vi "AI_ReadData.vi"(3 "error IO":errorcluster, 4 "count":i32, 6 "Task ID":u32) -> (0 "error out":errorcluster, 1 "data":dbl[](array[numeric]), 2 "Task ID":u32)   [LabVIEW 2015]
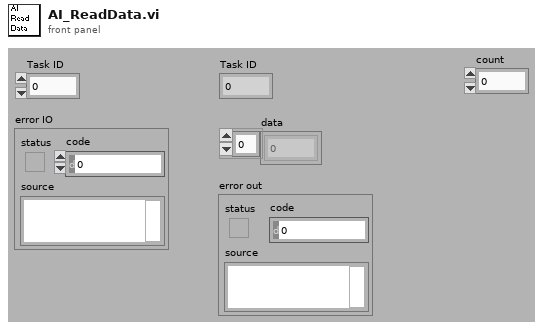
[diagram p1: front panel]
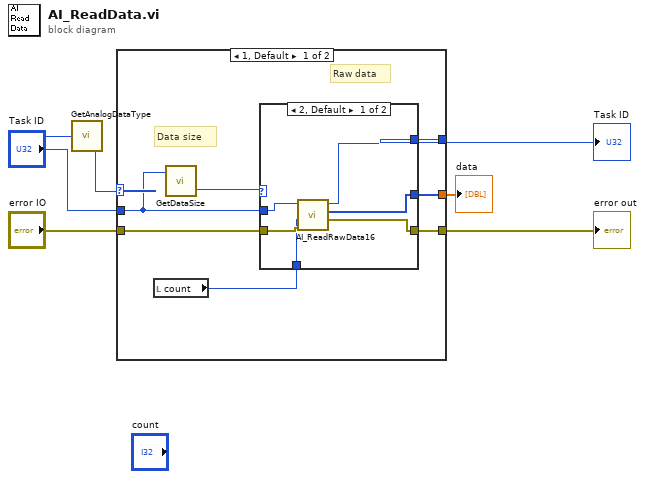
[diagram p0: block diagram]
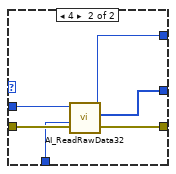
[diagram p2: hidden frame]
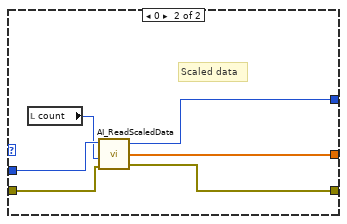
[diagram p3: hidden frame]
diagram:
  n1 = call "GetAnalogDataType.vi"("Task ID"="Task ID") -> ("return type"=w1:i32)
  n2 = case shown="1, Default" w1 {
    tunnel: "Task ID" -> [w8 w31]
    tunnel: "error IO" -> [w13 w30]
    tunnel: [w11 w29] -> w4
    tunnel: [w10 w27] -> w6
    tunnel: [w12 w28] -> w5
    frame 1, Default {
      # "Raw data"
      # "Data size"
      n3 = local read "count"() -> (w9:i32)
      n4 = call "GetDataSize.vi"("Task ID"=w8) -> ("return type"=w7:i32)  [unwired: 2 out]
      n5 = case shown="2, Default" w7 {
        tunnel: w13 -> [w18 w25]
        tunnel: [w17 w24] -> w12
        tunnel: [w16 w23] -> w11
        tunnel: w8 -> [w19 w22]
        tunnel: [w15 w21] -> w10
        tunnel: w9 -> [w14 w20]
        frame 2, Default {
          n6 = call "AI_ReadRawData16.vi"("Task ID"=w19, "count"=w14, "error in (no error)"=w18) -> ("Task ID"=w17:u32, "data"=w15:u16[], "error out"=w16:errorcluster)  [unwired: 1 in, 4 out]
        }
        frame 4 {
          n7 = call "AI_ReadRawData32.vi"("Task ID"=w22, "count"=w20, "error in (no error)"=w25) -> ("Task ID"=w24:u32, "data"=w21:u32[], "error out"=w23:errorcluster)  [unwired: 1 in, 4 out]
        }
      }
    }
    frame 0 {
      # "Scaled data"
      n8 = local read "count"() -> (w26:i32)
      n9 = call "AI_ReadScaledData.vi"("error in (no error)"=w30, "count"=w26, "Task ID"=w31) -> ("error out"=w29:errorcluster, "data"=w27:dbl[], "Task ID"=w28:u32)  [unwired: 1 in]
    }
  }
  "data" <- w6
  "Task ID" <- w5
  "error out" <- w4
